vi "2B TCP Packet.vi"(0 "ID":string, 5 "Version":string, 7 "utc_time":u32, 9 "PTP Sync":string="0", 11 "ue9LJ temp":u16, 12 "Flight Number":string, 13 "Data String":string) -> (8 "TCP Binary Packet":string)   [LabVIEW 2012]
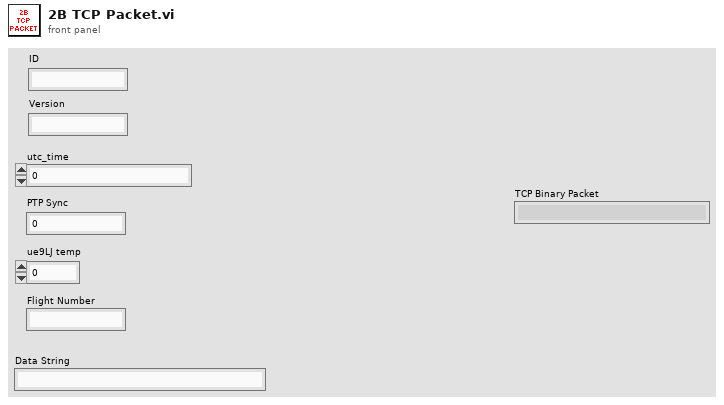
[diagram p1: front panel]
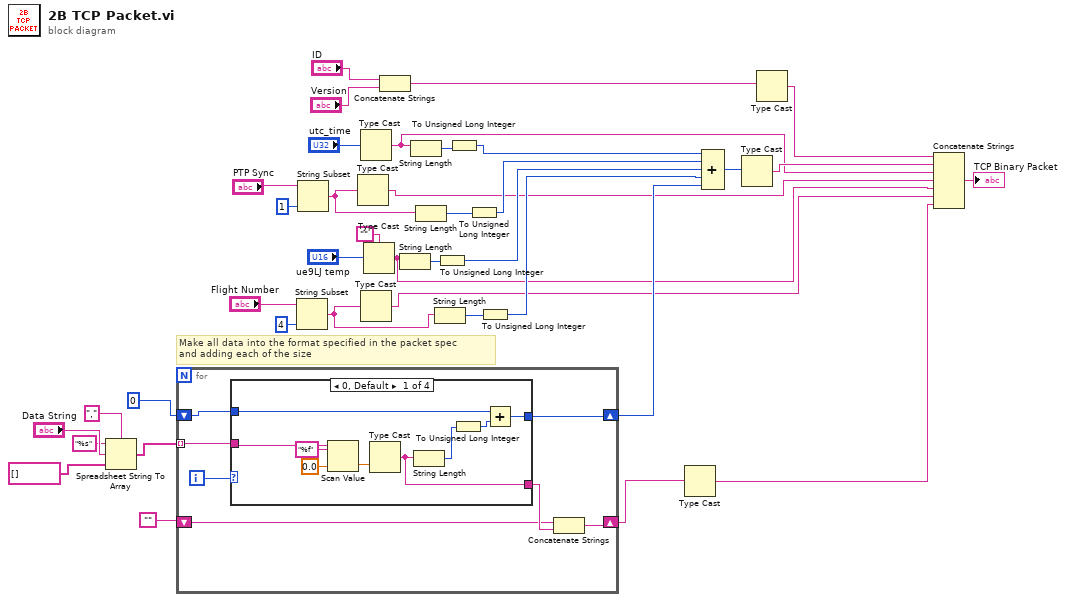
[diagram p0: block diagram]
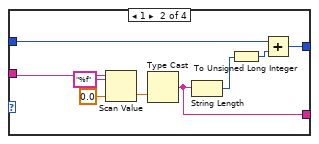
[diagram p2: hidden frame]
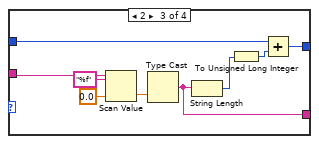
[diagram p3: hidden frame]
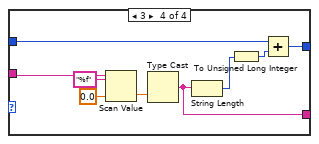
[diagram p4: hidden frame]
diagram:
  # "Make all data into the format specified in the packet spec\nand adding each of the size"
  n1 = Spreadsheet String To Array(delimiter (Tab)=",", format string="%s", spreadsheet string="Data String", array type (2D Dbl)=string[] []) -> (array=w1:string[])
  n2 = for {
    tunnel: w1 -> [w44] mode=indexing
    shift-right: [w42] -> w19
    shift-left: u32 0 -> [w43]
    shift-right: [w41] -> w6
    shift-left: "" -> [w39]
    i -> [w45]
    n3 = case shown="0, Default" w45 {
      tunnel: w44 -> [w52 w61 w70 w79]
      tunnel: w43 -> [w50 w59 w68 w77]
      tunnel: [w47 w56 w65 w74] -> w42
      tunnel: [w46 w55 w64 w73] -> w40
      frame 0, Default {
        n4 = Scan Value(string=w52, format string="%f", default (0 dbl)=sgl 0.0 ("default (0 I32)")) -> (value=w54:sgl)  [unwired: 1 out]
        n5 = Type Cast(x=w54) -> (*(type *) &x=w46:string)  [unwired: 1 in]
        n6 = String Length(string=w46) -> (length=w49:i32)
        n7 = To Unsigned Long Integer(number=w49) -> (unsigned 32bit integer=w48:u32)
        n8 = Add(x=w50, y=w48) -> (x+y=w47:u32)
      }
      frame 1 {
        n9 = Scan Value(string=w61, format string="%f", default (0 dbl)=sgl 0.0 ("default (0 I32)")) -> (value=w63:sgl)  [unwired: 1 out]
        n10 = Type Cast(x=w63) -> (*(type *) &x=w55:string)  [unwired: 1 in]
        n11 = String Length(string=w55) -> (length=w58:i32)
        n12 = To Unsigned Long Integer(number=w58) -> (unsigned 32bit integer=w57:u32)
        n13 = Add(x=w59, y=w57) -> (x+y=w56:u32)
      }
      frame 2 {
        n14 = Scan Value(string=w70, format string="%f", default (0 dbl)=sgl 0.0 ("default (0 I32)")) -> (value=w72:sgl)  [unwired: 1 out]
        n15 = Type Cast(x=w72) -> (*(type *) &x=w64:string)  [unwired: 1 in]
        n16 = String Length(string=w64) -> (length=w67:i32)
        n17 = To Unsigned Long Integer(number=w67) -> (unsigned 32bit integer=w66:u32)
        n18 = Add(x=w68, y=w66) -> (x+y=w65:u32)
      }
      frame 3 {
        n19 = Scan Value(string=w79, format string="%f", default (0 dbl)=sgl 0.0 ("default (0 I32)")) -> (value=w81:sgl)  [unwired: 1 out]
        n20 = Type Cast(x=w81) -> (*(type *) &x=w73:string)  [unwired: 1 in]
        n21 = String Length(string=w73) -> (length=w76:i32)
        n22 = To Unsigned Long Integer(number=w76) -> (unsigned 32bit integer=w75:u32)
        n23 = Add(x=w77, y=w75) -> (x+y=w74:u32)
      }
    }
    n24 = Concatenate Strings(w39, w40) -> (w41:string)
  }
  n25 = String Subset(string="Flight Number", length (rest)=4 ("length (rest)")) -> (substring=w10:string)  [unwired: 1 in]
  n26 = String Subset(string="PTP Sync", length (rest)=1 ("length (rest)")) -> (substring=w14:string)  [unwired: 1 in]
  n27 = Type Cast(x=w14) -> (*(type *) &x=w13:string)  [unwired: 1 in]
  n28 = Type Cast(x="utc_time") -> (*(type *) &x=w15:string)  [unwired: 1 in]
  n29 = Type Cast(x=w10) -> (*(type *) &x=w11:string)  [unwired: 1 in]
  n30 = Type Cast(type="", x="ue9LJ temp") -> (*(type *) &x=w12:string)
  n31 = Concatenate Strings("ID", "Version") -> (w36:string)
  n32 = String Length(string=w12) -> (length=w27:i32)
  n33 = String Length(string=w15) -> (length=w35:i32)
  n34 = String Length(string=w14) -> (length=w31:i32)
  n35 = String Length(string=w10) -> (length=w23:i32)
  n36 = To Unsigned Long Integer(number=w27) -> (unsigned 32bit integer=w25:u32)
  n37 = To Unsigned Long Integer(number=w35) -> (unsigned 32bit integer=w33:u32)
  n38 = To Unsigned Long Integer(number=w31) -> (unsigned 32bit integer=w29:u32)
  n39 = To Unsigned Long Integer(number=w23) -> (unsigned 32bit integer=w21:u32)
  n40 = Type Cast(x=w6) -> (*(type *) &x=w9:string)  [unwired: 1 in]
  n41 = Compound Arithmetic op=ADD(w33, w29, w25, w21, w19) -> (w17:u32)
  n42 = Type Cast(x=w17) -> (*(type *) &x=w16:string)  [unwired: 1 in]
  n43 = Type Cast(x=w36) -> (*(type *) &x=w18:string)  [unwired: 1 in]
  n44 = Concatenate Strings(w18, w16, w15, w13, w12, w11, w9) -> (→"TCP Binary Packet":string)
